vi "Load ASE Geometry.vi"(8 "error in (no error)":errorcluster, 11 "Model File":path) -> (0 "error out":errorcluster, 3 "New Mesh Refnum":refnum<vi>)   [LabVIEW 2020, in "NI_3D Picture Control.lvlib"]
doc: "Loads a three-dimensional object model saved in 3D Studio ASCII Exchange (ASE) format to display in a 3D scene."
uses:
  <vilib>/picture/3D Picture Control/NI_3D Picture Control.lvlib
  <vilib>/picture/3D Picture Control/NI_Old 3D Toolkit.lvlib
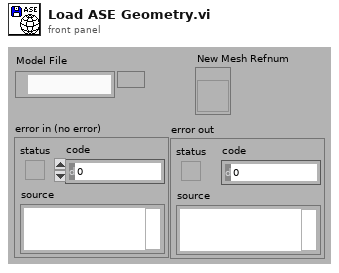
[diagram p1: front panel]
types:
  T1 = enum16{"Z -> Y  &  -Y -> Z", "X -> Z  &  -Z -> X", "Y -> X  &  -X -> Y", "None"}
  T2 = typedef "NI_3D Picture Control.lvlib/NI_Old 3D Toolkit.lvlib/model.ctl" = cluster{"VertexList":T3[], "FaceList":cluster{"v1":i32, "v2":i32, "v3":i32}[], "NormalList":T3[], "Mode":T4}
  T3 = typedef "NI_3D Picture Control.lvlib/NI_Old 3D Toolkit.lvlib/point3f.ctl" = cluster{"x":sgl, "y":sgl, "z":sgl}
  T4 = typedef "NI_3D Picture Control.lvlib/NI_Old 3D Toolkit.lvlib/VertexMode.ctl" = enum16{"GL_POINTS", "GL_LINES", "GL_LINE_LOOP", "GL_LINE_STRIP", "GL_TRIANGLES", "GL_TRIANGLE_STRIP", "GL_TRIANGLE_FAN", "GL_QUADS", "GL_QUAD_STRIP", "GL_POLYGON"}
  T5 = enum16{"Points", "Lines", "Line Strip", "Line Loop", "Triangles", "Triangle Strip", "Triangle Fan", "Quads", "Quad Strip", "Polygon"}
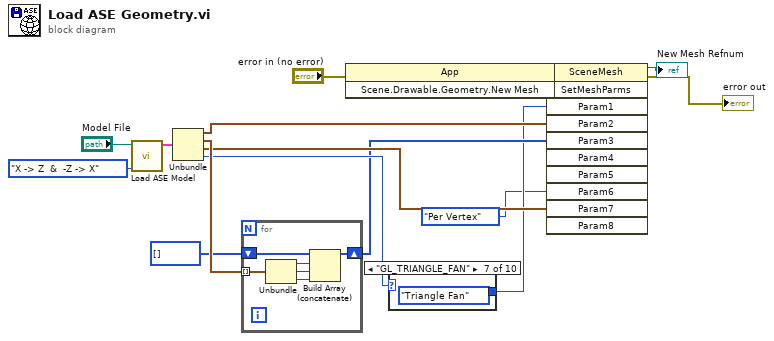
[diagram p0: block diagram]
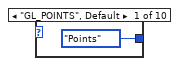
[diagram p2: hidden frame]
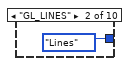
[diagram p3: hidden frame]
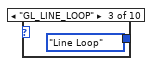
[diagram p4: hidden frame]
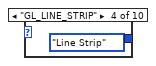
[diagram p5: hidden frame]
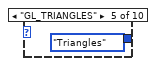
[diagram p6: hidden frame]
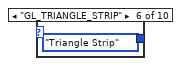
[diagram p7: hidden frame]
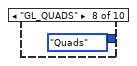
[diagram p8: hidden frame]
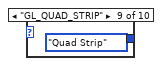
[diagram p9: hidden frame]
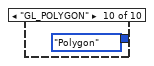
[diagram p10: hidden frame]
diagram:
  n1 = call <vilib>:"Load ASE Model.vi"("Normal Correction"=T1."X -> Z  &  -Z -> X", "Model File"="Model File") -> ("Model"=w16:T2)  [unwired: 9 in]
  n2 = Unbundle(w16) -> ("VertexList"=w5:T3[], "FaceList"=w15:cluster{"v1":i32, "v2":i32, "v3":i32}[], "NormalList"=w4:T3[], "Mode"=w13:T4)
  n3 = for {
    tunnel: w15 -> [w22] mode=indexing
    shift-right: [w18] -> w3
    shift-left: i32[] [] -> [w17]
    n4 = Unbundle(w22) -> ("v1"=w21:i32, "v2"=w20:i32, "v3"=w19:i32)
    n5 = Build Array (concatenate)(w17, w21, w20, w19) -> (w18:i32[])
  }
  n6 = invoke class="App" method="Scene.Drawable.Geometry.New Mesh"(error in="error in (no error)") -> (error out=w10:errorcluster, "Scene.Geometry.New Mesh"=w12:refnum<vi>)  [unwired: 2 in, 1 out]
  n7 = case shown="\"GL_TRIANGLE_FAN\"" w13 {
    tunnel: [T5."Points" ("Draw Mode") T5."Lines" ("Draw Mode") T5."Line Loop" ("Draw Mode") T5."Line Strip" ("Draw Mode") T5."Triangles" ("Draw Mode") T5."Triangle Strip" ("Draw Mode") T5."Triangle Fan" ("Draw Mode") T5."Quads" ("Draw Mode") T5."Quad Strip" ("Draw Mode") T5."Polygon" ("Draw Mode")] -> w2
    frame "GL_POINTS", Default {
    }
    frame "GL_LINES" {
    }
    frame "GL_LINE_LOOP" {
    }
    frame "GL_LINE_STRIP" {
    }
    frame "GL_TRIANGLES" {
    }
    frame "GL_TRIANGLE_STRIP" {
    }
    frame "GL_TRIANGLE_FAN" {
    }
    frame "GL_QUADS" {
    }
    frame "GL_QUAD_STRIP" {
    }
    frame "GL_POLYGON" {
    }
  }
  n8 = invoke class="SceneMesh" method="SetMeshParms"(reference=w12, error in=w10, "Param1"=w2, "Param2"=w5, "Param3"=w3, "Param6"=enum16{"Overall", "Per Primitive", "Per Vertex"}."Per Vertex" ("Normal Binding Mode"), "Param7"=w4) -> (reference out=→"New Mesh Refnum":refnum<vi>, error out=→"error out":errorcluster)  [unwired: 4 in, 9 out]
